vi "kinfe edge method.vi"(0 "Speed":cluster{"Speed":i32, "Vi":i32, "Vi steps":i32}={"Speed"=8000, "Vi"=1000, "Vi steps"=800} {"Speed" min=50 max=8000 step=50 scale=50.0..8000.0}, 1 "Go_stop":bool, 2 "PosCtrl":T2={"Go x"=FALSE, "Back x"=FALSE, "Go y"=FALSE, "Back y"=FALSE, "Go z"=FALSE, "Back z"=FALSE, "dX (um)"=1000, "dY (um)"=0, "dZ (um)"=0} {"dX (um)" step=1}, 5 "Home":bool, 7 "Zero":bool, 10 "stop 2":bool, 11 "VISA resource (RS232)":refnum<visa-resource-name>="COM1") -> (3 "?":cluster{"X":dbl, "Y":dbl, "Z":dbl}, 9 "Static":bool)   [LabVIEW 2014]
uses:
  <vilib>/vision/driver/NI_Vision_Acquisition_Software.lvlib
  <vilib>/Instr/_visa.llb/VISA Configure Serial Port (Instr).vi
  <vilib>/userdefined/High Color/IMAQdx.ctl
panel:
  out "um/s":string
  out "um(x) 2":string
  out "um(y)":string
  out "appended array":dbl[](array[numeric])
  out "fitting (y&T)":dbl[][](array[numeric])
  out "path (for logistic)":path
  out "row data save path":path
  in  "cluster":cluster{"T&Y(output)":dbl[][], "dt":dbl} {"dt" format="%#_13g"}
  out "T&Y(output)":dbl[][](array[numeric])
  out "Y(output)":dbl[](array[numeric])
  out "T(output)":dbl[](array[numeric])
  out "Initial X":dbl format="%^.3e"
  out "X Increment":dbl format="%^.3e"
  out "Y(all)":dbl[](array[numeric]) caption="Waveform Array" format="%^.3e"
  out "T(all)":dbl[](array[numeric])
  in  "Tout":i32
  in  "timeout":i32=5000 caption="Timeout\n[ms]"
  out "Waveform":T1(graph)
  out "Acquisitions":i32
  in  "Tab Control 2":enum32{"MAIN", "knife edge method", "Setting"}(tab)
  in  "?":enum32{" RS232", "ESP32"}(tab)
  in  "x-":bool caption="Start"
  in  "x+":bool caption="Start"
  out "um(x)":string
  in  "y+":bool caption="Start"
  in  "y-":bool caption="Start"
  in  "um":i32
  in  "um":i32
  in  "Channel":i32[](array[ring]) caption="Channel (1)" items=["1"=1, "2"=2, "3"=3, "4"=4, "off"=0]
  in  "?":bool
  in  "Get Image":bool
  out "Snap Image":T3(plugin-control)
  out "Grab Image":T3(plugin-control)
  in  "?":T4(tab)
  out "waveform 1":cluster{"T":dbl[], "Waveform Array":dbl[]}(graph)
  in  "unit":u16(ring) items=["s"=0, "ms"=3, "us"=6, "ns"=9]
  out "test read":dbl[](array[numeric])
  out "times":i32
  out "row data1":dbl[](array[numeric])
  out "row data1 2":dbl[](array[numeric])
  in  "Paramter guess":dbl[](array[numeric])=[-4.2, 0.0, 100.0, 1.0, 1.0]
  out "output cluster 2":T5
  out "waveform 2":cluster{"T":dbl[], "Waveform Array":dbl[]}(graph)
  in  "Save data":bool caption="Fitting"
  out "output cluster":T6
  in  "Slide":cluster{dbl, dbl}(slide)={0.0, 1.2121212121212122} scale=-0.9999920000000001..1.0000059999741622
  in  "name":string
  in  "Path":path
  out "XY Graph":cluster{cdb[]}[](graph)
  out "E":i32
  in  "fitting(Logistic)":bool caption="Fitting"
  in  "save(Logistic)":bool caption="Fitting"
  out "point":i32
  out "waveform 1":cluster{"T":dbl[], "Waveform Array":dbl[]}(graph)
  out "Samples count":i32[](array[numeric])
  in  "Exit":bool
  in  "Stop":bool
  in  "Single":bool
  in  "Start":bool
  out "ActiveChannels":i32[](array[numeric])=[1, 4]
  in  "channel on":i32=1 min=1 max=4 step=1
  in  "speed(um/s)":i32
  in  "move(um)":i32
  in  "knife edge method":bool caption="Start"
  in  "knife edge method(stop)":bool caption="Start"
  in  "VISA resource name 2":refnum<visa-resource-name>="TCPIP0::169.254.236.131::inst0::INSTR" caption="VISA resource name"
  in  "VISA resource name":refnum<visa-resource-name>="TCPIP::169.254.236.131::HISLIP"
  out "Moving Time (Sec)":dbl
  in  "VISA resource (esp32)":refnum<visa-resource-name>="COM8"
  in  "Delay (ms)":u32=100
  in  "update period (ms)":u32=100
  in  "Go":bool
  in  "Back":bool
  in  "X0":T7 {"Y (um)" min=0.0; "X (um)" min=0.0}
  in  "Scaling":cluster{"X":u16, "Y":u16, "Z":u16} {"Z" items=["X", "Z", "None"]; "Y" items=["X", "Z", "None"]; "X" items=["X", "Z", "None"]}
  in  "Position to go":T8={"Position"={"X"=FALSE, "Target X (um)"=1000.0, "Current X (um)"=1000.0, "Scaling X"=0, "Y"=FALSE, "Target Y (um)"=0.0, "Current Y (um)"=0.0, "Scaling Y"=0, "Z"=FALSE, "Target Z (um)"=0.0, "Current Z (um)"=0.0, "Scaling Z"=0}, "Speed"={"Speed"=3111, "Vi steps"=800, "Vi"=1000}} {"Speed"."Speed" min=50 max=8000 step=50 scale=50.0..8000.0; "Position"."Current X (um)" step=1.0; "Position"."Scaling Z" items=["X", "Z", "None"]; "Position"."Scaling Y" items=["X", "Z", "None"]; "Position"."Scaling X" items=["X", "Z", "None"]; "Position"."Target X (um)" step=1.0}
  in  "Camera COM":T9
  out "Position Info":T10={"Current coordinates"={"Steps"=0.0, "X"=FALSE, "Steps 2"=0.0, "Y"=FALSE, "Steps 3"=0.0, "Z"=FALSE}, "read buffer"="", "Command"="a", "Current coordinates 2"={"X"=0.0, "Y"=0.0, "Z"=0.0}, "Moving Time (Sec)"=0.0}
  out "RS232 error":errorcluster
  # "Only For Knife Edge Method"
  # "y0\n\nx0\n\nK\n\nL\n\nA"
  # "Esp32"
  # "CCD"
  # "RTO"
  # "RS232"
  # "Origin"
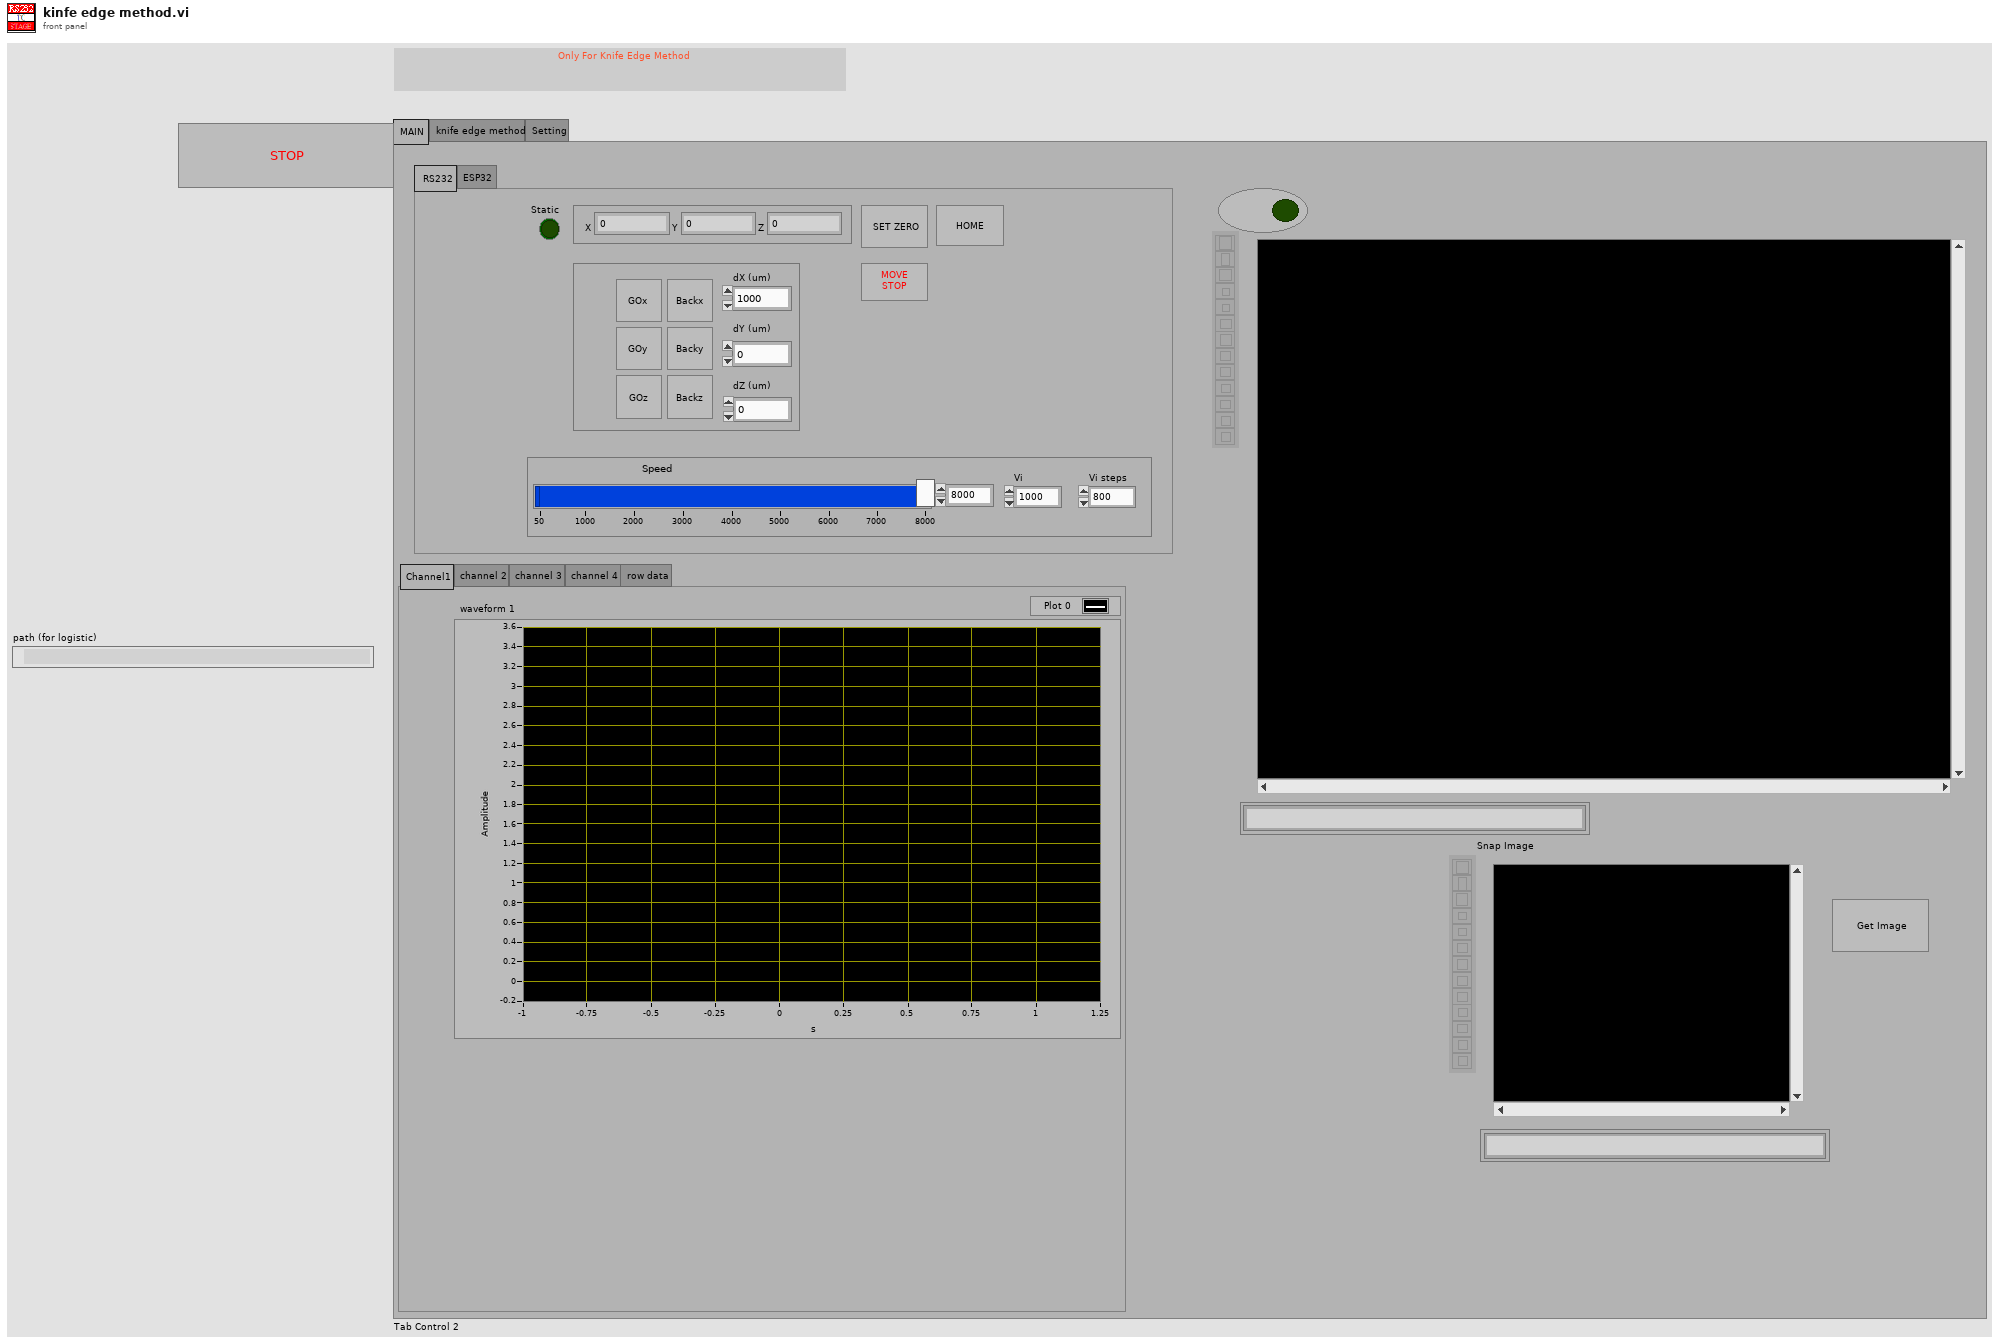
[diagram p1: front panel]
types:
  T1 = cluster{"Initial X":dbl, "X Increment":dbl, "Waveform Array":dbl[]}[]
  T2 = cluster{"Go x":bool, "Back x":bool, "Go y":bool, "Back y":bool, "Go z":bool, "Back z":bool, "dX (um)":u32, "dY (um)":u32, "dZ (um)":u32}
  T3 = typedef "IMAQ Image.ctl" = refnum<image>
  T4 = enum32{"Channel1", "channel 2", "channel 3", "channel 4", "row data"}
  T5 = cluster{"y0":dbl, "x0":dbl, "best fit parameters":dbl[]}
  T6 = cluster{"T(all)":dbl[], "Y(all)":dbl[], "X Increment":dbl, "Initial X":dbl}
  T7 = cluster{"X (um)":dbl, "X 2":bool, "Y (um)":dbl, "Y 2":bool, "Z (um)":dbl, "Z 2":bool}
  T8 = cluster{"Position":cluster{"X":bool, "Target X (um)":dbl, "Current X (um)":dbl, "Scaling X":u16, "Y":bool, "Target Y (um)":dbl, "Current Y (um)":dbl, "Scaling Y":u16, "Z":bool, "Target Z (um)":dbl, "Current Z (um)":dbl, "Scaling Z":u16}, "Speed":cluster{"Speed":i32, "Vi steps":i32, "Vi":i32}}
  T9 = typedef "IMAQdx.ctl" = refnum<k21>
  T10 = cluster{"Current coordinates":cluster{"Steps":dbl, "X":bool, "Steps 2":dbl, "Y":bool, "Steps 3":dbl, "Z":bool}, "read buffer":string, "Command":string, "Current coordinates 2":cluster{"X":dbl, "Y":dbl, "Z":dbl}, "Moving Time (Sec)":dbl}
  T11 = cluster{"X":bool, "Target X (um)":dbl, "Current X (um)":dbl, "Scaling X":u16, "Y":bool, "Target Y (um)":dbl, "Current Y (um)":dbl, "Scaling Y":u16, "Z":bool, "Target Z (um)":dbl, "Current Z (um)":dbl, "Scaling Z":u16}
  T12 = cluster{"Go x":bool, "Back x":bool, "Go y":bool, "Back y":bool, "Go z":bool, "Back z":bool, "dX (um)":dbl, "dY (um)":dbl, "dZ (um)":dbl}
  T13 = cluster{"Position":cluster{"X":bool, "Target X (um)":dbl, "Current X (um)":dbl, "Scaling X":u16, "Y":bool, "Target Y (um)":dbl, "Current Y (um)":dbl, "Scaling Y":u16, "Z":bool, "Target Z (um)":dbl, "Current Z (um)":dbl, "Scaling Z":u16}, "Value":cluster{"Speed":i32, "Vi":i32, "Vi steps":i32}}
  T14 = cluster{"Task":u16, cluster{"Position":cluster{"X":bool, "Target X (um)":dbl, "Current X (um)":dbl, "Scaling X":u16, "Y":bool, "Target Y (um)":dbl, "Current Y (um)":dbl, "Scaling Y":u16, "Z":bool, "Target Z (um)":dbl, "Current Z (um)":dbl, "Scaling Z":u16}, "Value":cluster{"Speed":i32, "Vi":i32, "Vi steps":i32}}}
  T15 = cluster{"Task":u16, "Position to go":cluster{"Position":cluster{"X":bool, "Target X (um)":dbl, "Current X (um)":dbl, "Scaling X":u16, "Y":bool, "Target Y (um)":dbl, "Current Y (um)":dbl, "Scaling Y":u16, "Z":bool, "Target Z (um)":dbl, "Current Z (um)":dbl, "Scaling Z":u16}, "Speed":cluster{"Speed":i32, "Vi steps":i32, "Vi":i32}}}
  T16 = cluster{"Task 2":u16, "Position to go 2":cluster{"Position":cluster{"X":bool, "Target X (um)":dbl, "Current X (um)":dbl, "Scaling X":u16, "Y":bool, "Target Y (um)":dbl, "Current Y (um)":dbl, "Scaling Y":u16, "Z":bool, "Target Z (um)":dbl, "Current Z (um)":dbl, "Scaling Z":u16}, "Speed":cluster{"Speed":i32, "Vi steps":i32, "Vi":i32}}}
  T17 = cluster{"Go x":bool, "Back x":bool, "Go y":bool, "Back y":bool, "Go z":bool, "Back z":bool, "dX (um)":bool, "dY (um)":bool, "dZ (um)":bool}
  T18 = cluster{"Initial X":dbl, "X Increment":dbl, "Waveform Array":dbl[]}
  T19 = cluster{"Ring":u16, "Value":cluster{"Position":cluster{"X":bool, "Target X (um)":dbl, "Current X (um)":dbl, "Scaling X":u16, "Y":bool, "Target Y (um)":dbl, "Current Y (um)":dbl, "Scaling Y":u16, "Z":bool, "Target Z (um)":dbl, "Current Z (um)":dbl, "Scaling Z":u16}, "Speed":cluster{"Speed":i32, "Vi steps":i32, "Vi":i32}}}
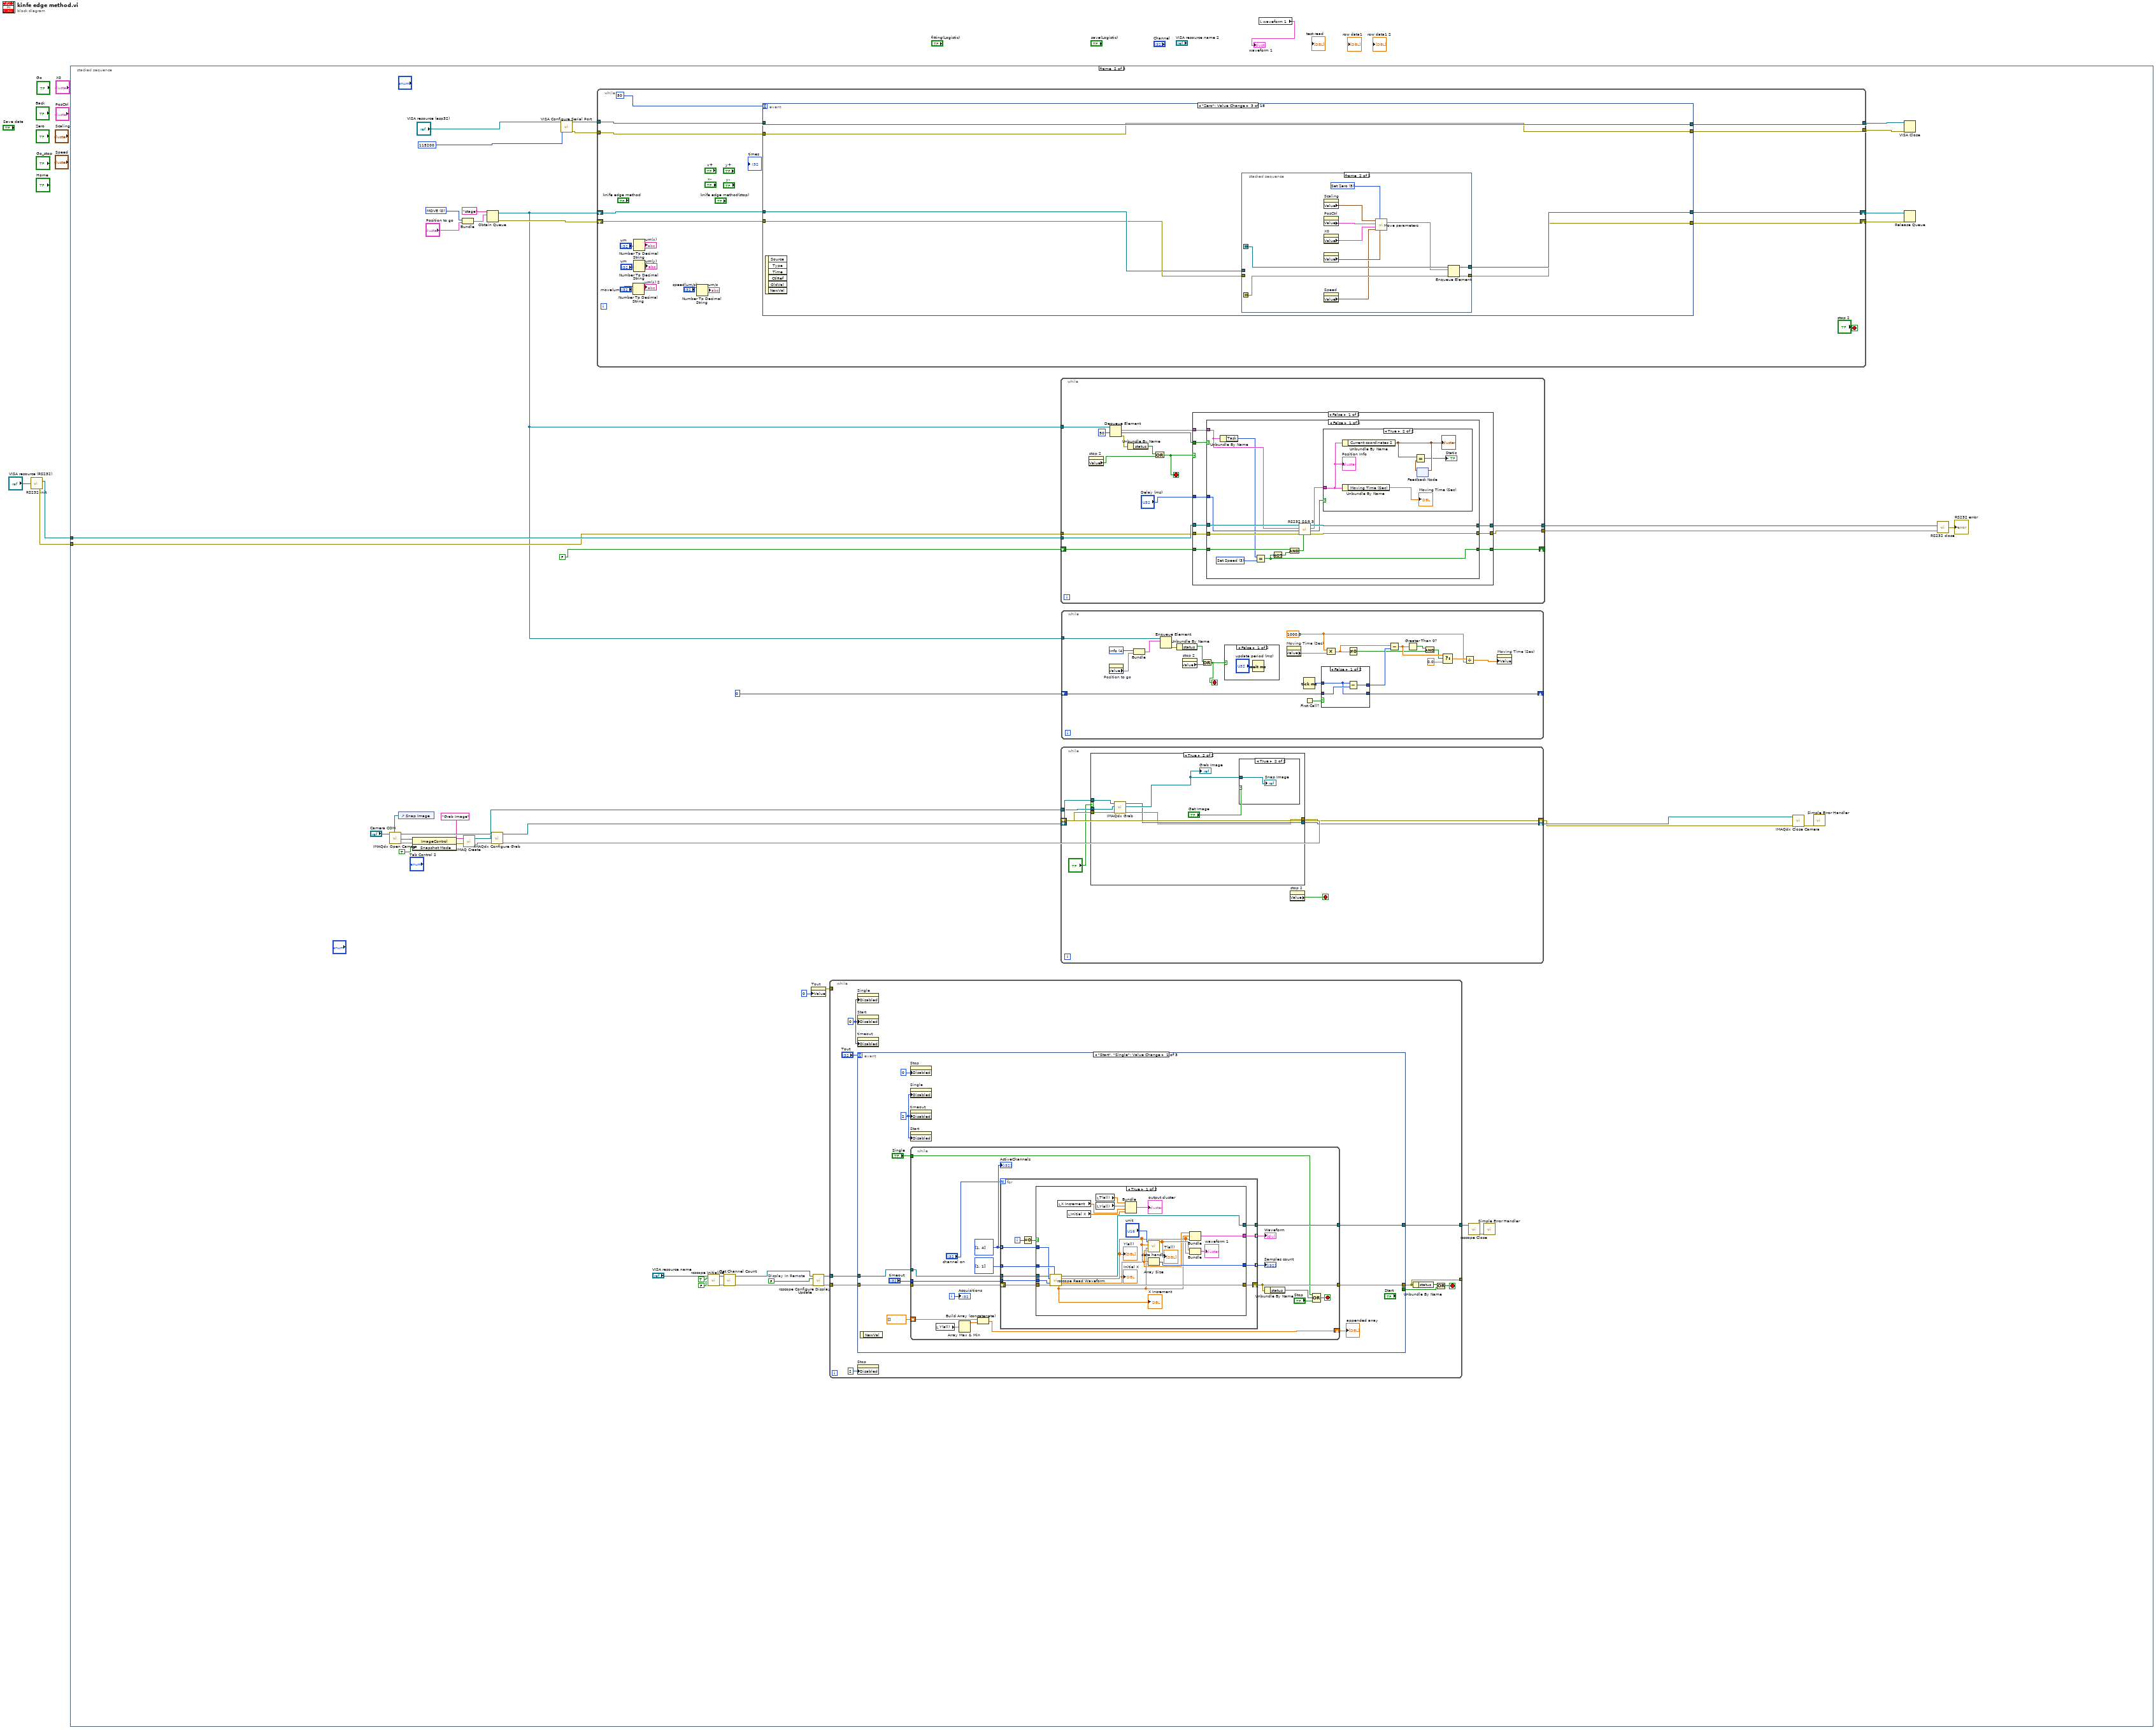
[diagram p0: block diagram]
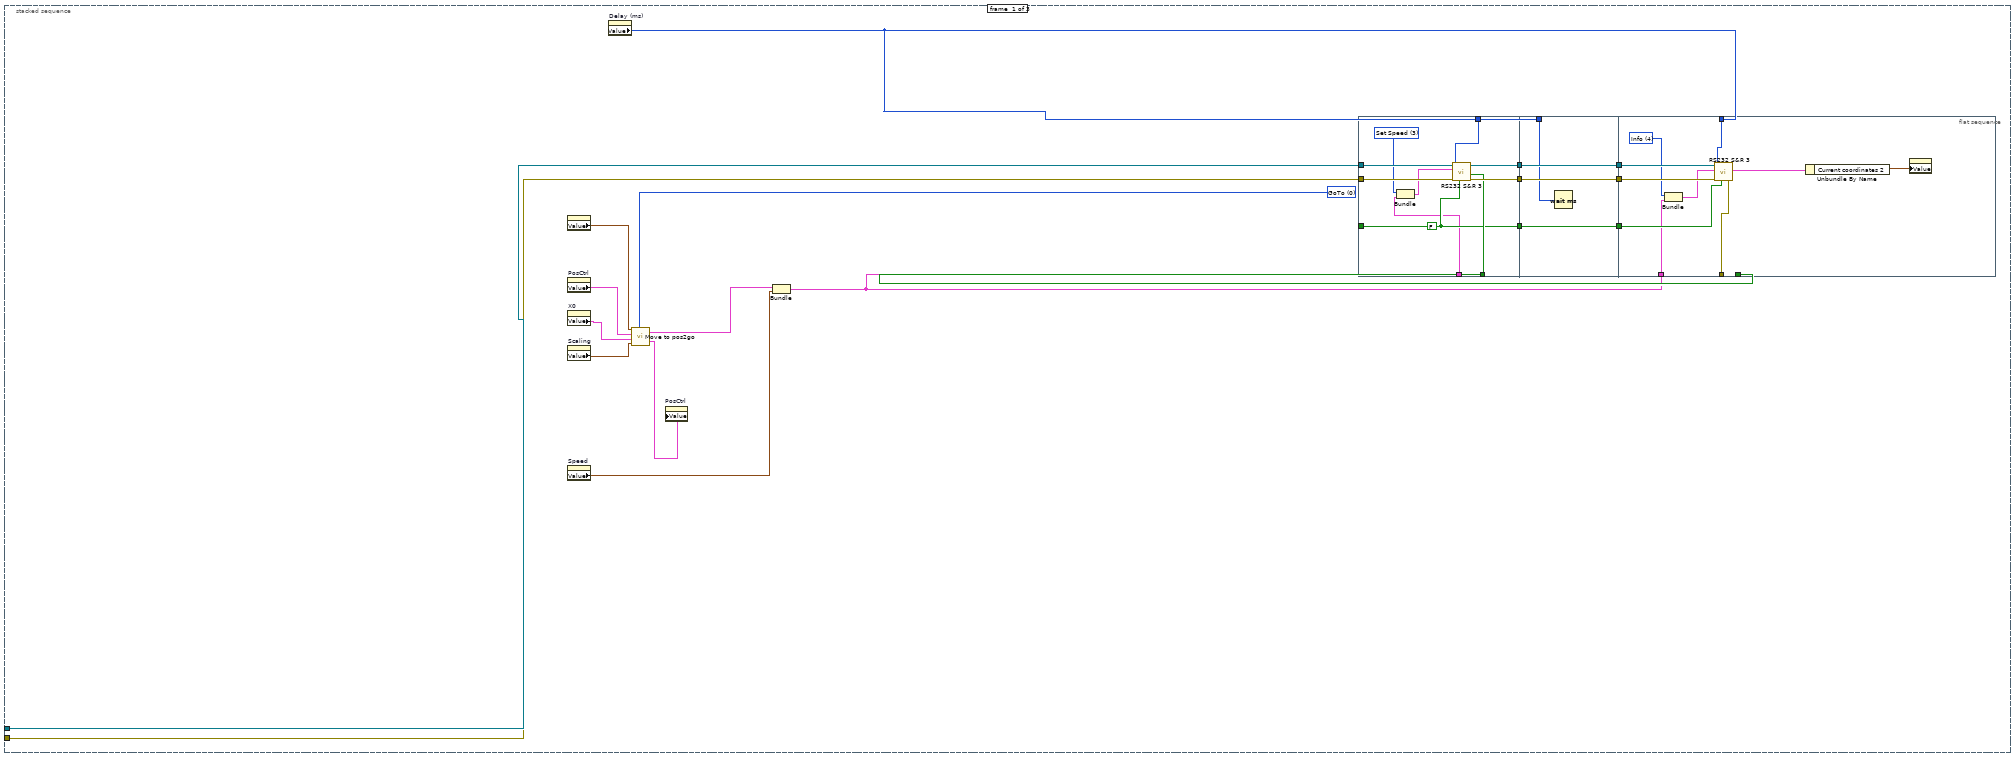
[diagram p2: hidden frame]
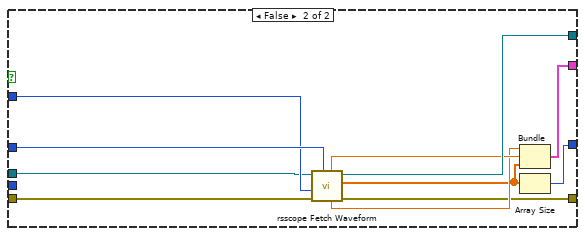
[diagram p3: hidden frame]
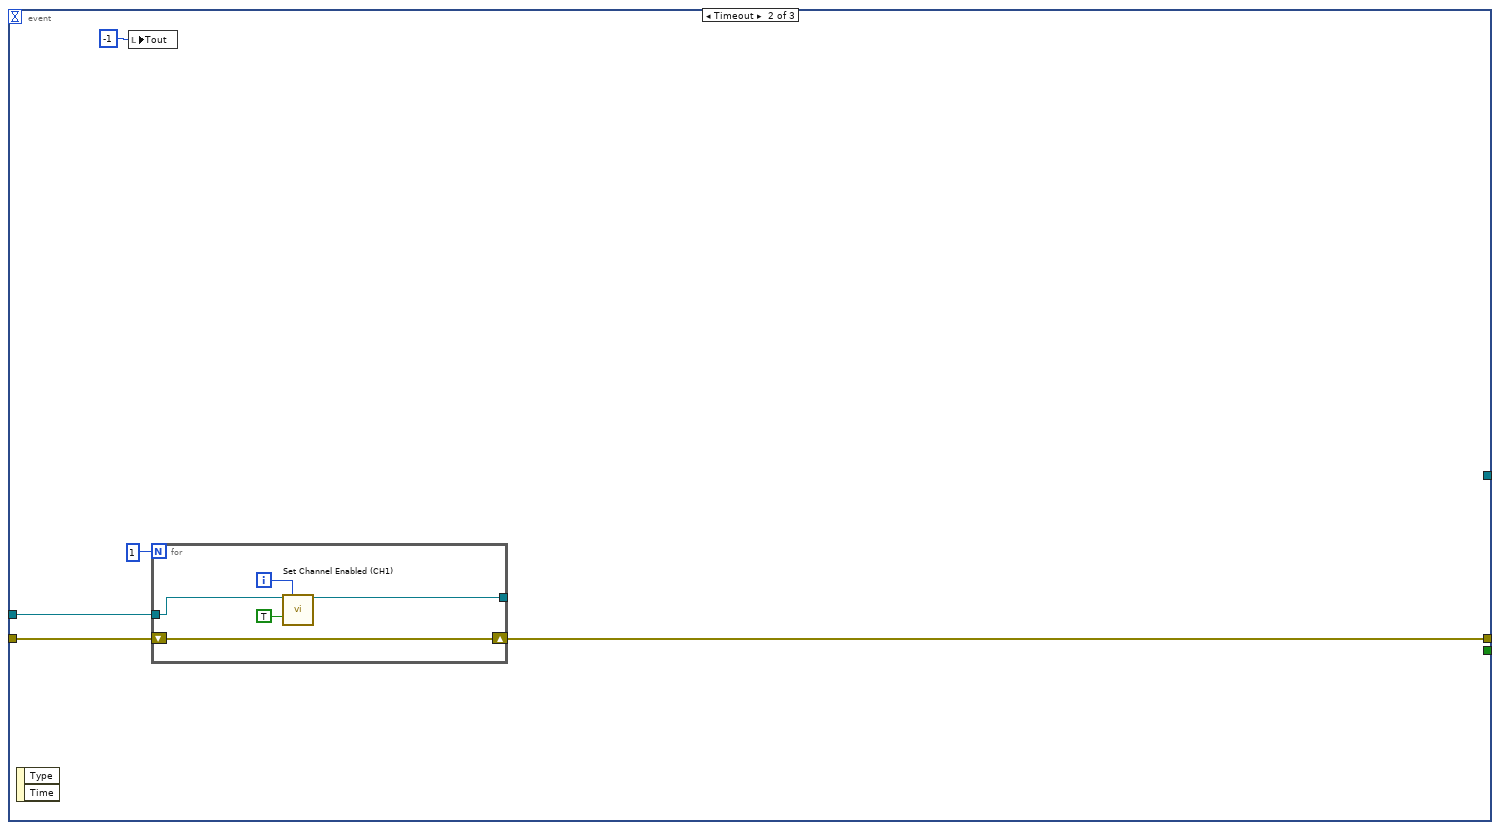
[diagram p4: hidden frame]
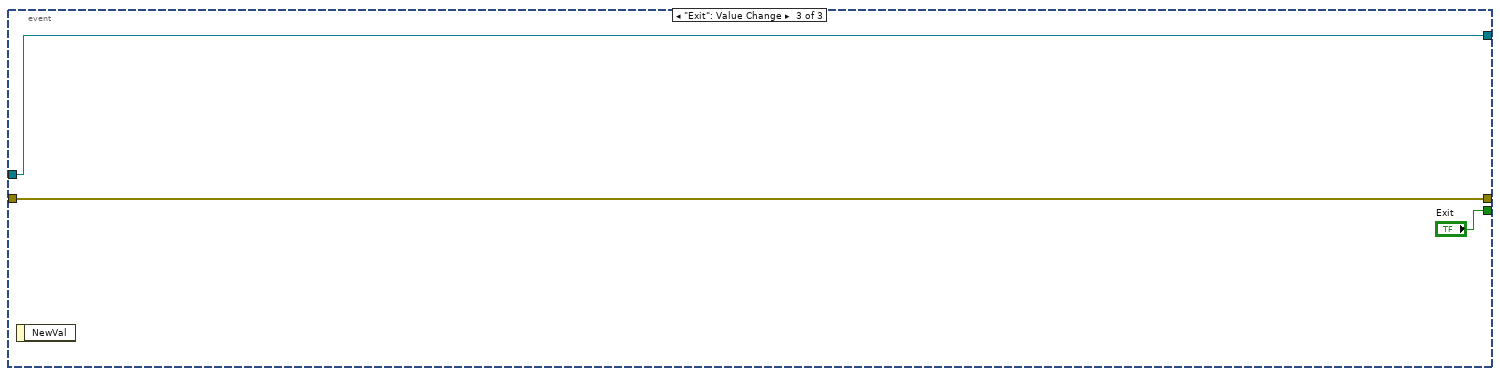
[diagram p5: hidden frame]
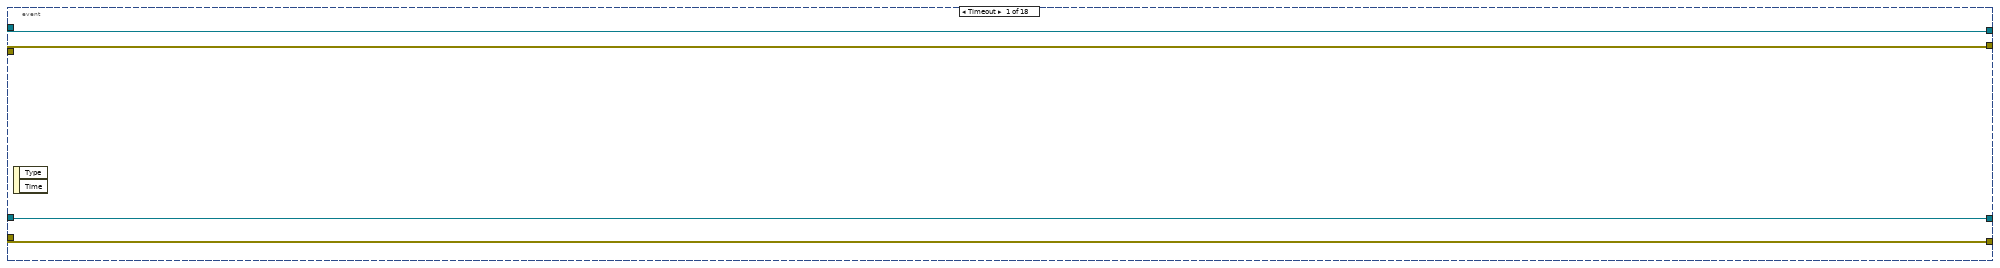
[diagram p13: hidden frame]
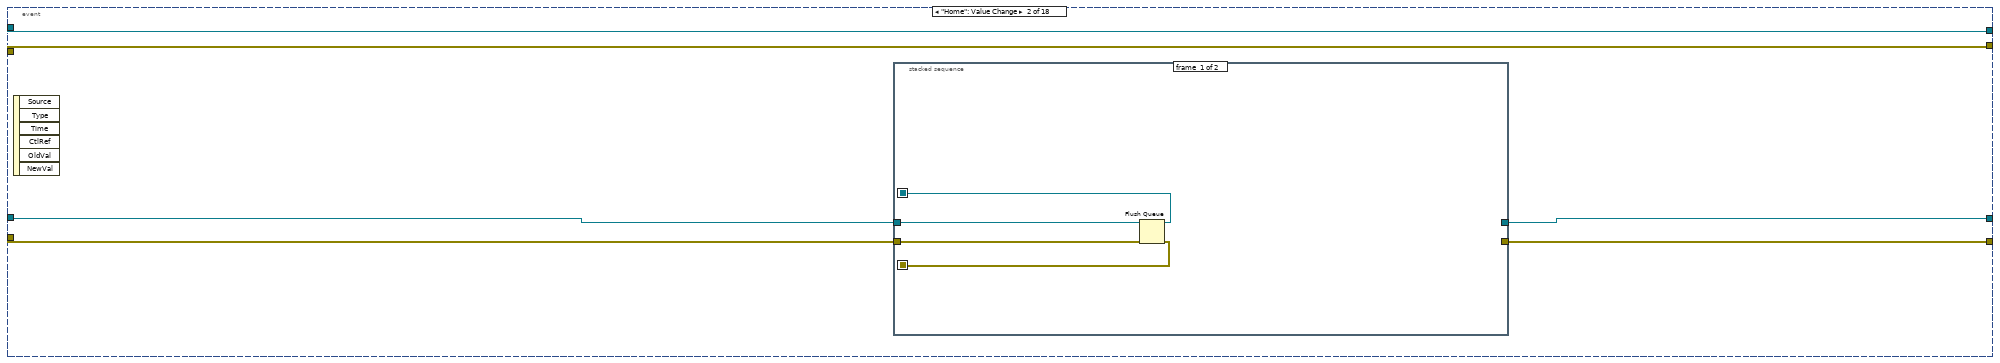
[diagram p14: hidden frame]
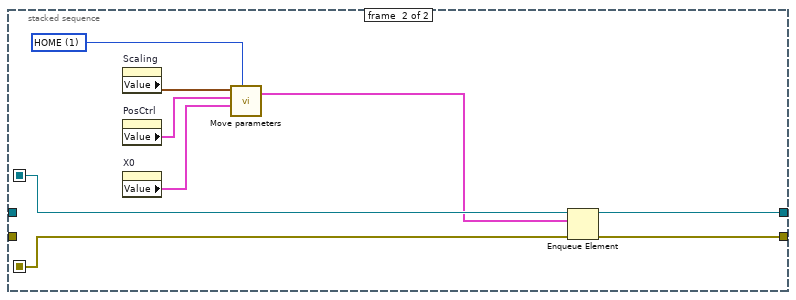
[diagram p15: hidden frame]
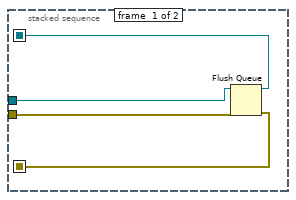
[diagram p16: hidden frame]
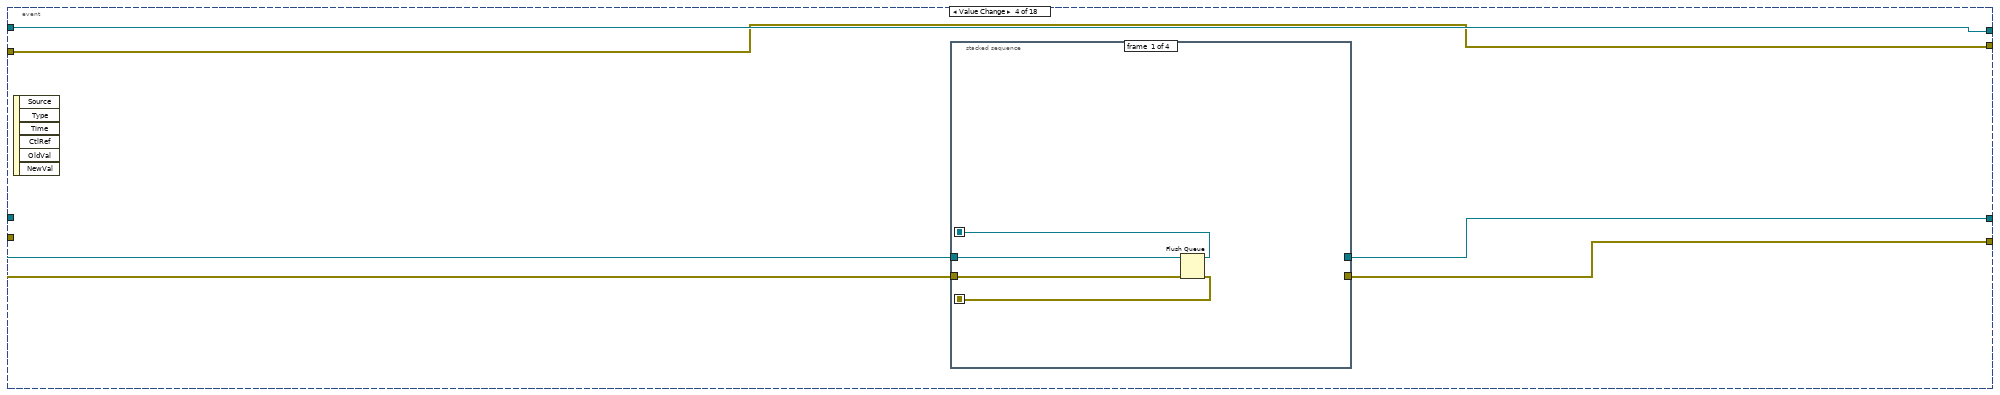
[diagram p17: hidden frame]
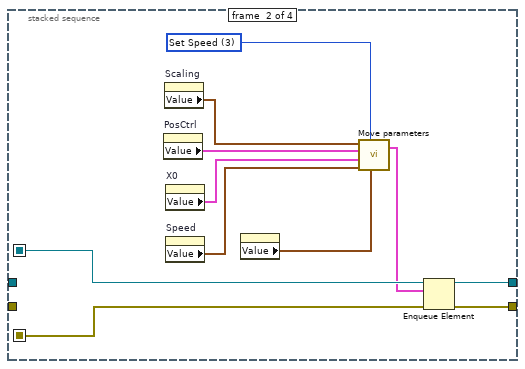
[diagram p18: hidden frame]
diagram:
  n1 = call "RS232 init.vi"("VISA resource name"="VISA resource (RS232)") -> ("VISA resource name out"=w3:refnum<visa-resource-name>, "error out"=w2:errorcluster)
  n2 = stacked-sequence {
    tunnel: w3 -> [w6 w90 _]
    tunnel: w2 -> [w5 w89 _]
    frame #0 {
      w11 = u16 0 items=["GoTo", "Jog"] ("Mode")
      n3 = property class="Clust (strict)"() -> ("Value"=w14:cluster{"X":dbl, "Y":dbl, "Z":dbl})  [unwired: 2 in, 2 out]
      n4 = property on="PosCtrl" class="Clust (strict)"() -> ("Value"=w13:T2)  [unwired: 2 in, 2 out]
      n5 = property on="X0" class="Clust (strict)"() -> ("Value"=w7:T7)  [unwired: 2 in, 2 out]
      n6 = property on="Scaling" class="Clust (strict)"() -> ("Value"=w12:cluster{"X":u16, "Y":u16, "Z":u16})  [unwired: 2 in, 2 out]
      n7 = property on="Speed" class="Clust (strict)"() -> ("Value"=w9:cluster{"Speed":i32, "Vi":i32, "Vi steps":i32})  [unwired: 2 in, 2 out]
      n8 = property on="Delay (ms)" class="DigNum (strict)"() -> ("Value"=w18:u32)  [unwired: 2 in, 2 out]
      n9 = call "Move to pos2go.vi"("Current coordinates"=w14, "DelX"=w13, "X0"=w7, "Scaling"=w12, "Mode"=w11) -> ("Position"=w10:T11, "DelX 2"=w8:T12)
      n10 = property on="PosCtrl" class="Clust (strict)"("Value"=w8) -> ()  [unwired: 2 in, 2 out]
      n11 = Bundle("Position"=w10, "Value"=w9) -> (w15:T13)  [unwired: 1 in]
      n12 = flat-sequence {
        tunnel: w6 -> [w34]
        tunnel: w5 -> [w33]
        tunnel: [w29] -> w16
        tunnel: w15 -> [w26]
        tunnel: [w32] -> w24
        tunnel: [w31] -> w23
        tunnel: w18 -> [w30]
        tunnel: FALSE -> [w28]
        tunnel: [w28] -> w22
        tunnel: [w38] -> w21
        tunnel: w24 -> [w38]
        tunnel: [w37] -> w20
        tunnel: w23 -> [w37]
        tunnel: w18 -> [w36]
        tunnel: [w35] -> w19
        tunnel: w22 -> [w35]
        tunnel: w21 -> [w48]
        tunnel: w20 -> [w47]
        tunnel: w18 -> [w46]
        tunnel: [w44] -> _
        tunnel: w16 -> [_]
        tunnel: w19 -> [w43]
        tunnel: w15 -> [w41]
        frame #0 {
          w27 = u16 3 items=["MOVE", "HOME", "STOP", "Set Speed", "Info", "Set Zero"] ("Task")
          n13 = Bundle("Task"=w27, w26) -> (w25:T14)  [unwired: 1 in]
          n14 = call "RS232 S&R 3.vi"("ReSetSPD"=w28, "error in"=w33, "Delay (ms)"=w30, "Stage Control"=w25, "VISA resource in"=w34) -> ("error out"=w31:errorcluster, "read"=w29:bool, "VISA resource name out"=w32:refnum<visa-resource-name>)  [unwired: 1 out]
        }
        frame #1 {
          n15 = Wait (ms)(milliseconds to wait=w36) -> ()  [unwired: 1 out]
        }
        frame #2 {
          w40 = u16 4 items=["MOVE", "HOME", "STOP", "Set Speed", "Info", "Set Zero"] ("Task")
          n16 = Bundle("Task"=w40, w41) -> (w39:T14)  [unwired: 1 in]
          n17 = call "RS232 S&R 3.vi"("ReSetSPD"=w43, "error in"=w47, "Delay (ms)"=w46, "Stage Control"=w39, "VISA resource in"=w48) -> ("error out"=w44:errorcluster, "Cluster"=w42:T10)  [unwired: 2 out]
          n18 = Unbundle By Name(w42) -> ("Current coordinates 2"=w45:cluster{"X":dbl, "Y":dbl, "Z":dbl})
          n19 = property class="Clust (strict)"("Value"=w45) -> ()  [unwired: 2 in, 2 out]
        }
      }
    }
    frame #1 {
      w55 = FALSE  # Display In Remote
      w95 = u16 0 items=["MOVE", "HOME", "STOP", "Set Speed", "Info", "Set Zero", "MOVE2"] ("Task")
      n20 = call <vilib>:"IMAQdx Open Camera.vi"("Session In"="Camera COM") -> ("error out"=w75:errorcluster, "Session Out"=w74:T9)  [unwired: 2 in, 7 out]
      n21 = control-ref of="Snap Image"() -> (w76:refnum<vi>)
      n22 = property class="ImageControl"(reference=w76, error in=w75, "Snapshot Mode"=TRUE) -> (error out=w73:errorcluster)  [unwired: 1 out]
      n23 = Bundle("Task"=w95, "Position to go"="Position to go") -> (w96:T15)  [unwired: 1 in]
      n24 = call "IMAQ Create"("Image Name"="Grab Image", "error in (no error)"=w73) -> ("New Image"=w63:T3, "error out"=w72:errorcluster)  [unwired: 2 in, 1 out]
      n25 = Obtain Queue(name (unnamed)="stage", element data type=w96) -> (queue out=w84:refnum<queue>, error out=w93:errorcluster)  [unwired: 3 in, 1 out]
      n26 = call <vilib>:"IMAQdx Configure Grab.vi"("error in"=w72, "Session In"=w74) -> ("error out"=w65:errorcluster, "Session Out"=w64:T9)  [unwired: 8 out]
      n27 = call-poly "VISA Configure Serial Port"("VISA resource name"="VISA resource (esp32)", "baud rate (9600)"=u32 115200) -> ("VISA resource name out"=w80:refnum<visa-resource-name>, "error out"=w79:errorcluster)  [unwired: 12 in]
      n28 = while {
        shift-right: [w301] -> w92
        shift-left: w84 -> [w304]
        shift-right: [w300] -> w91
        shift-left: w93 -> [w303]
        tunnel: w80 -> [w287]
        tunnel: w79 -> [w288]
        tunnel: [w299] -> w78
        tunnel: [w298] -> w77
        stop <- "stop 2" stop-if-true
        n29 = Number To Decimal String(number="move(um)") -> (decimal integer string=→"um(x) 2":string)  [unwired: 1 in]
        n30 = Number To Decimal String(number="um") -> (decimal integer string=→"um(x)":string)  [unwired: 1 in]
        n31 = Number To Decimal String(number="um") -> (decimal integer string=→"um(y)":string)  [unwired: 1 in]
        n32 = Number To Decimal String(number="speed(um/s)") -> (decimal integer string=→"um/s":string)  [unwired: 1 in]
        n33 = event shown="[2] \"Zero\": Value Change" {
          selector: _ -> [_ _ _ _ _ _ _ _ _ _ _ _ _ _ _ _ _ _]
          dyn-events: _ -> [_ _ _ _ _ _ _ _ _ _ _ _ _ _ _ _ _ _]
          timeout: 50 -> [_ _ _ _ _ _ _ _ _ _ _ _ _ _ _ _ _ _]
          tunnel: w304 -> [w308 w314 w333 w354 w375 w396 w417 w438 w481 w495 w503 w514 w522 w532 w542 w553 w564 w574]
          tunnel: w303 -> [w307 w313 w332 w353 w374 w395 w416 w437 w480 w494 w502 w513 w521 w531 w541 w552 w563 w573]
          tunnel: [w308 w312 w331 w352 w373 w394 w415 w436 w481 w495 w503 w514 w522 w532 w542 w553 w564 w574] -> w301
          tunnel: [w307 w311 w330 w351 w372 w393 w414 w435 w480 w494 w502 w513 w521 w531 w541 w552 w563 w573] -> w300
          tunnel: w287 -> [w306 w310 w329 w350 w371 w392 w413 w434 w483 w497 w505 w516 w526 w536 w546 w557 w568 w576]
          tunnel: w288 -> [w305 w309 w328 w349 w370 w391 w412 w433 w482 w496 w504 w515 w525 w535 w545 w556 w567 w575]
          tunnel: [w306 w310 w329 w350 w371 w392 w413 w434 w483 w497 w505 w516 w524 w534 w544 w555 w562 w572] -> w299
          tunnel: [w305 w309 w328 w349 w370 w391 w412 w433 w482 w496 w504 w515 w523 w533 w543 w554 w561 w571] -> w298
          event Timeout {
            n34 = event-data() -> ()  [unwired: 1 in, 2 out]
          }
          event "Home": Value Change {
            n35 = event-data() -> ()  [unwired: 1 in, 6 out]
            n36 = stacked-sequence {
              seq-local: [w315 _] -> [_ w325]
              seq-local: [w316 _] -> [_ w324]
              tunnel: w314 -> [w318 _]
              tunnel: w313 -> [w317 _]
              tunnel: [_ w327] -> w312
              tunnel: [_ w326] -> w311
              frame #0 {
                n37 = Flush Queue(queue=w318, error in (no error)=w317) -> (queue out=w315:refnum<queue>, error out=w316:errorcluster)  [unwired: 1 out]
              }
              frame #1 {
                w320 = u16 1 items=["MOVE", "HOME", "ZERO", "Set speed", "Info"] ("Ring")
                n38 = property on="Scaling" class="Clust (strict)"() -> ("Value"=w323:cluster{"X":u16, "Y":u16, "Z":u16})  [unwired: 2 in, 2 out]
                n39 = property on="PosCtrl" class="Clust (strict)"() -> ("Value"=w322:T2)  [unwired: 2 in, 2 out]
                n40 = property on="X0" class="Clust (strict)"() -> ("Value"=w319:T7)  [unwired: 2 in, 2 out]
                n41 = call "Move parameters.vi"("Task"=w320, "X0"=w319, "PosCtrl"=w322, "Scaling"=w323) -> ("Move info"=w321:T16)  [unwired: 2 in, 1 out]
                n42 = Enqueue Element(queue=w325, element=w321, error in (no error)=w324) -> (queue out=w327:refnum<queue>, error out=w326:errorcluster)  [unwired: 1 in, 1 out]
              }
            }
          }
          event "Zero": Value Change {
            n43 = event-data() -> ()  [unwired: 1 in, 6 out]
            n44 = stacked-sequence {
              seq-local: [w335 _] -> [_ w348]
              seq-local: [w336 _] -> [_ w347]
              tunnel: w332 -> [w337 _]
              tunnel: [_ w346] -> w331
              tunnel: [_ w345] -> w330
              tunnel: w333 -> [w334 _]
              frame #0 {
                n45 = Flush Queue(queue=w334, error in (no error)=w337) -> (queue out=w335:refnum<queue>, error out=w336:errorcluster)  [unwired: 1 out]
              }
              frame #1 {
                w344 = u16 5 items=["MOVE", "HOME", "STOP", "Set Speed", "Info", "Set Zero"] ("Task")
                n46 = property on="Scaling" class="Clust (strict)"() -> ("Value"=w342:cluster{"X":u16, "Y":u16, "Z":u16})  [unwired: 2 in, 2 out]
                n47 = property on="PosCtrl" class="Clust (strict)"() -> ("Value"=w341:T2)  [unwired: 2 in, 2 out]
                n48 = property on="X0" class="Clust (strict)"() -> ("Value"=w340:T7)  [unwired: 2 in, 2 out]
                n49 = property class="Clust (strict)"() -> ("Value"=w343:cluster{"X":dbl, "Y":dbl, "Z":dbl})  [unwired: 2 in, 2 out]
                n50 = property on="Speed" class="Clust (strict)"() -> ("Value"=w339:cluster{"Speed":i32, "Vi":i32, "Vi steps":i32})  [unwired: 2 in, 2 out]
                n51 = call "Move parameters.vi"("Current coordinates"=w343, "Task"=w344, "Speed"=w339, "X0"=w340, "PosCtrl"=w341, "Scaling"=w342) -> ("Move info"=w338:T16)  [unwired: 1 out]
                n52 = Enqueue Element(queue=w348, element=w338, error in (no error)=w347) -> (queue out=w346:refnum<queue>, error out=w345:errorcluster)  [unwired: 1 in, 1 out]
              }
            }
          }
          event "Speed.Speed": Value Change {
            n53 = event-data() -> ()  [unwired: 1 in, 6 out]
            n54 = stacked-sequence {
              seq-local: [w356 _ _ _] -> [_ w367 _ _]
              seq-local: [w355 _ _ _] -> [_ w366 _ _]
              tunnel: w354 -> [w358 _ _ _]
              tunnel: [_ w369 _ _] -> w352
              tunnel: w353 -> [w357 _ _ _]
              tunnel: [_ w368 _ _] -> w351
              frame #0 {
                n55 = Flush Queue(queue=w358, error in (no error)=w357) -> (queue out=w356:refnum<queue>, error out=w355:errorcluster)  [unwired: 1 out]
              }
              frame #1 {
                w365 = u16 3 items=["MOVE", "HOME", "STOP", "Set Speed", "Info", "Set Zero"] ("Task")
                n56 = property on="PosCtrl" class="Clust (strict)"() -> ("Value"=w363:T2)  [unwired: 2 in, 2 out]
                n57 = property on="Scaling" class="Clust (strict)"() -> ("Value"=w364:cluster{"X":u16, "Y":u16, "Z":u16})  [unwired: 2 in, 2 out]
                n58 = property on="X0" class="Clust (strict)"() -> ("Value"=w362:T7)  [unwired: 2 in, 2 out]
                n59 = property on="Speed" class="Clust (strict)"() -> ("Value"=w361:cluster{"Speed":i32, "Vi":i32, "Vi steps":i32})  [unwired: 2 in, 2 out]
                n60 = property class="Clust (strict)"() -> ("Value"=w360:cluster{"X":dbl, "Y":dbl, "Z":dbl})  [unwired: 2 in, 2 out]
                n61 = call "Move parameters.vi"("Current coordinates"=w360, "Task"=w365, "Speed"=w361, "X0"=w362, "PosCtrl"=w363, "Scaling"=w364) -> ("Move info"=w359:T16)  [unwired: 1 out]
                n62 = Enqueue Element(queue=w367, element=w359, error in (no error)=w366) -> (queue out=w369:refnum<queue>, error out=w368:errorcluster)  [unwired: 1 in, 1 out]
              }
              frame #2 {
              }
              frame #3 {
              }
            }
          }
          event "Go": Value Change {
            n63 = event-data() -> ()  [unwired: 1 in, 6 out]
            n64 = stacked-sequence {
              seq-local: [w376 _] -> [_ w388]
              seq-local: [w377 _] -> [_ w387]
              tunnel: w375 -> [w379 _]
              tunnel: w374 -> [w378 _]
              tunnel: [_ w390] -> w373
              tunnel: [_ w389] -> w372
              frame #0 {
                n65 = Flush Queue(queue=w379, error in (no error)=w378) -> (queue out=w376:refnum<queue>, error out=w377:errorcluster)  [unwired: 1 out]
              }
              frame #1 {
                w380 = u16 6 items=["MOVE", "HOME", "STOP", "Set Speed", "Info", "Set Zero", "MOVE2"] ("Task")
                n66 = property on="Scaling" class="Clust (strict)"() -> ("Value"=w384:cluster{"X":u16, "Y":u16, "Z":u16})  [unwired: 2 in, 2 out]
                n67 = property on="PosCtrl" class="Clust (strict)"() -> ("Value"=w385:T2)  [unwired: 2 in, 2 out]
                n68 = property on="X0" class="Clust (strict)"() -> ("Value"=w383:T7)  [unwired: 2 in, 2 out]
                n69 = property on="Speed" class="Clust (strict)"() -> ("Value"=w382:cluster{"Speed":i32, "Vi":i32, "Vi steps":i32})  [unwired: 2 in, 2 out]
                n70 = property class="Clust (strict)"() -> ("Value"=w381:cluster{"X":dbl, "Y":dbl, "Z":dbl})  [unwired: 2 in, 2 out]
                n71 = call "Move parameters.vi"("Current coordinates"=w381, "Task"=w380, "Speed"=w382, "X0"=w383, "PosCtrl"=w385, "Scaling"=w384) -> ("Move info"=w386:T16)  [unwired: 1 out]
                n72 = Enqueue Element(queue=w388, element=w386, error in (no error)=w387) -> (queue out=w390:refnum<queue>, error out=w389:errorcluster)  [unwired: 1 in, 1 out]
              }
            }
          }
          event "Back": Value Change {
            n73 = event-data() -> ()  [unwired: 1 in, 6 out]
            n74 = stacked-sequence {
              seq-local: [w397 _] -> [_ w409]
              seq-local: [w398 _] -> [_ w408]
              tunnel: w396 -> [w400 _]
              tunnel: w395 -> [w399 _]
              tunnel: [_ w411] -> w394
              tunnel: [_ w410] -> w393
              frame #0 {
                n75 = Flush Queue(queue=w400, error in (no error)=w399) -> (queue out=w397:refnum<queue>, error out=w398:errorcluster)  [unwired: 1 out]
              }
              frame #1 {
                w401 = u16 6 items=["MOVE", "HOME", "STOP", "Set Speed", "Info", "Set Zero", "MOVE2"] ("Task")
                n76 = property on="Scaling" class="Clust (strict)"() -> ("Value"=w405:cluster{"X":u16, "Y":u16, "Z":u16})  [unwired: 2 in, 2 out]
                n77 = property on="PosCtrl" class="Clust (strict)"() -> ("Value"=w406:T2)  [unwired: 2 in, 2 out]
                n78 = property on="X0" class="Clust (strict)"() -> ("Value"=w404:T7)  [unwired: 2 in, 2 out]
                n79 = property on="Speed" class="Clust (strict)"() -> ("Value"=w403:cluster{"Speed":i32, "Vi":i32, "Vi steps":i32})  [unwired: 2 in, 2 out]
                n80 = property class="Clust (strict)"() -> ("Value"=w402:cluster{"X":dbl, "Y":dbl, "Z":dbl})  [unwired: 2 in, 2 out]
                n81 = call "Move parameters.vi"("Current coordinates"=w402, "Task"=w401, "Speed"=w403, "X0"=w404, "PosCtrl"=w406, "Scaling"=w405) -> ("Move info"=w407:T16)  [unwired: 1 out]
                n82 = Enqueue Element(queue=w409, element=w407, error in (no error)=w408) -> (queue out=w411:refnum<queue>, error out=w410:errorcluster)  [unwired: 1 in, 1 out]
              }
            }
          }
          event "Go_stop": Value Change {
            n83 = event-data() -> ()  [unwired: 1 in, 6 out]
            n84 = stacked-sequence {
              seq-local: [w418 _] -> [_ w429]
              seq-local: [w419 _] -> [_ w430]
              tunnel: w417 -> [w421 _]
              tunnel: w416 -> [w420 _]
              tunnel: [_ w432] -> w415
              tunnel: [_ w431] -> w414
              frame #0 {
                n85 = Flush Queue(queue=w421, error in (no error)=w420) -> (queue out=w418:refnum<queue>, error out=w419:errorcluster)  [unwired: 1 out]
              }
              frame #1 {
                w428 = u16 2 items=["MOVE", "HOME", "STOP", "Set Speed", "Info", "Set Zero"] ("Task")
                n86 = property on="Scaling" class="Clust (strict)"() -> ("Value"=w427:cluster{"X":u16, "Y":u16, "Z":u16})  [unwired: 2 in, 2 out]
                n87 = property on="PosCtrl" class="Clust (strict)"() -> ("Value"=w426:T2)  [unwired: 2 in, 2 out]
                n88 = property on="X0" class="Clust (strict)"() -> ("Value"=w425:T7)  [unwired: 2 in, 2 out]
                n89 = property on="Speed" class="Clust (strict)"() -> ("Value"=w424:cluster{"Speed":i32, "Vi":i32, "Vi steps":i32})  [unwired: 2 in, 2 out]
                n90 = property class="Clust (strict)"() -> ("Value"=w423:cluster{"X":dbl, "Y":dbl, "Z":dbl})  [unwired: 2 in, 2 out]
                n91 = call "Move parameters.vi"("Current coordinates"=w423, "Task"=w428, "Speed"=w424, "X0"=w425, "PosCtrl"=w426, "Scaling"=w427) -> ("Move info"=w422:T16)  [unwired: 1 out]
                n92 = Enqueue Element(queue=w429, element=w422, error in (no error)=w430) -> (queue out=w432:refnum<queue>, error out=w431:errorcluster)  [unwired: 1 in, 1 out]
              }
            }
          }
          event "PosCtrl": Value Change {
            n93 = event-data() -> ("OldVal"=w441:T2, "NewVal"=w440:T2)  [unwired: 1 in, 4 out]
            n94 = Equal?(x=w441, y=w440) -> (x = y?=w448:T17)
            n95 = Unbundle By Name(w448) -> ("Go x"=w447:bool, "Back x"=w446:bool, "Go y"=w445:bool, "Back y"=w444:bool, "Go z"=w443:bool, "Back z"=w442:bool)
            n96 = Compound Arithmetic op=OR(w447, w446, w445, w444, w443, w442) -> (w439:bool)
            n97 = case shown="True" w439 {
              tunnel: [w450 w454] -> w436
              tunnel: [w449 w453] -> w435
              tunnel: w438 -> [w450 w452]
              tunnel: w437 -> [w449 w451]
              frame False {
              }
              frame True {
                n98 = stacked-sequence {
                  seq-local: [w455 _ _] -> [_ w467 _]
                  seq-local: [w456 _ _] -> [_ w468 _]
                  seq-local: [_ w459 _] -> [_ _ w471]
                  tunnel: w452 -> [w458 _ _]
                  tunnel: w451 -> [w457 _ _]
                  tunnel: [_ w470 _] -> w454
                  tunnel: [_ w469 _] -> w453
                  frame #0 {
                    n99 = Flush Queue(queue=w458, error in (no error)=w457) -> (queue out=w455:refnum<queue>, error out=w456:errorcluster)  [unwired: 1 out]
                  }
                  frame #1 {
                    w460 = u16 0 items=["MOVE", "HOME", "STOP", "Set Speed", "Info", "Set Zero", "MOVE2"] ("Task")
                    n100 = property on="Scaling" class="Clust (strict)"() -> ("Value"=w466:cluster{"X":u16, "Y":u16, "Z":u16})  [unwired: 2 in, 2 out]
                    n101 = property on="PosCtrl" class="Clust (strict)"() -> ("Value"=w465:T2)  [unwired: 2 in, 2 out]
                    n102 = property on="X0" class="Clust (strict)"() -> ("Value"=w464:T7)  [unwired: 2 in, 2 out]
                    n103 = property on="Speed" class="Clust (strict)"() -> ("Value"=w463:cluster{"Speed":i32, "Vi":i32, "Vi steps":i32})  [unwired: 2 in, 2 out]
                    n104 = property class="Clust (strict)"() -> ("Value"=w462:cluster{"X":dbl, "Y":dbl, "Z":dbl})  [unwired: 2 in, 2 out]
                    n105 = call "Move parameters.vi"("Current coordinates"=w462, "Task"=w460, "Speed"=w463, "X0"=w464, "PosCtrl"=w465, "Scaling"=w466) -> ("PosCtrl out"=w459:T12, "Move info"=w461:T16)
                    n106 = Enqueue Element(queue=w467, element=w461, error in (no error)=w468) -> (queue out=w470:refnum<queue>, error out=w469:errorcluster)  [unwired: 1 in, 1 out]
                  }
                  frame #2 {
                    n107 = property on="PosCtrl" class="Clust (strict)"("Value"=w471) -> ()  [unwired: 2 in, 2 out]
                  }
                }
              }
            }
          }
          event "Slide": Value Change {
            n108 = event-data() -> ()  [unwired: 1 in, 6 out]
            n109 = local read "T&Y(output)"() -> (w475:dbl[][])
            n110 = local read "X Increment"() -> (w477:dbl)
            n111 = Transpose 2D Array(2D array=w475) -> (transposed array=w474:dbl[][])
            n112 = Bundle(w474, "X Increment"=w477) -> (w476:cluster{dbl[][], "X Increment":dbl})  [unwired: 1 in]
            n113 = local read "output cluster"() -> (w492:T6)
            n114 = local write "cluster"(w476) -> ()
            n115 = Unbundle(w492) -> ("T(all)"=w491:dbl[], "Y(all)"=w490:dbl[], "X Increment"=w488:dbl, "Initial X"=w489:dbl)
            n116 = call "split data.vi"("Slide"="Slide", "dt"=w488, "t0"=w489, "Y(input)"=w490, "T(input)"=w491) -> ("max value"=w485:dbl, "min value"=w486:dbl, "Y(output)"=w473:dbl[], "T(output)"=w479:dbl[])  [unwired: 2 in]
            "T(output)" <- w479
            "Y(output)" <- w473
            n117 = property on="Slide" class="Slide (strict)"("Scale.Maximum"=w485, "Scale.Minimum"=w486) -> ()  [unwired: 2 in, 2 out]
            n118 = Bundle("T(output)"=w479, "Y(output)"=w473) -> (→"waveform 2":cluster{"T(output)":dbl[], "Y(output)":dbl[]})  [unwired: 1 in]
            n119 = Array Size(array=w473) -> (size(s)=→"point":i32)
            n120 = Build Array(w479, w473) -> (→"T&Y(output)":dbl[][])
          }
          event "Save data": Value Change {
            n121 = event-data() -> ()  [unwired: 1 in, 6 out]
            n122 = call "save data.vi"("name"="name", "Path"="Path", "cluster"="cluster") -> ("new file path (Not A Path if cancelled)"=→"row data save path":path, "path(FOR logistic"=→"path (for logistic)":path)  [unwired: 6 in, 1 out]
          }
          event "fitting(Logistic)": Value Change {
            n123 = event-data() -> ()  [unwired: 1 in, 6 out]
            n124 = local read "Y(output)"() -> (w511:dbl[])
            n125 = local read "T(output)"() -> (w512:dbl[])
            n126 = call "Fittinglogistic_MODCA.vi"("Paramter guess"="Paramter guess", "y"=w511, "t"=w512) -> ("fitting (y&T)"=→"fitting (y&T)":dbl[][], "E"=→"E":i32, "XY Graph"=→"XY Graph":cluster{cdb[]}[], "output cluster"=→"output cluster 2":T5)  [unwired: 5 in]
          }
          event "save(Logistic)": Value Change {
            n127 = event-data() -> ()  [unwired: 1 in, 6 out]
            n128 = local read "path (for logistic)"() -> (w517:path)
            n129 = local read "fitting (y&T)"() -> (w518:dbl[][])
            n130 = local read "Paramter guess"() -> (w520:dbl[])
            n131 = call "logistic save.vi"("file path (dialog if empty)"=w517, "format (%.3f)"="%.7e", "Paramter guess"=w520, "2D data"=w518) -> ()  [unwired: 10 in, 2 out]
          }
          event "x+": Value Change {
            w530 = u16 1 items=["Move X"=1, "Move Y"=2, "Single shot"=3, "single shot *15"=4, "energy adjustment"=5, "knife edge method"=6, "Auto mode"=7] ("Ring")
            n132 = event-data() -> ()  [unwired: 1 in, 6 out]
            n133 = local read "um(x)"() -> (w528:string)
            n134 = call "0814 labviewToEsp32.vi"("direction"="0", "um"=w528, "Ring"=w530) -> ("output"=w527:string)  [unwired: 8 in]
            n135 = VISA Write(VISA resource name=w526, write buffer=w527, error in (no error)=w525) -> (VISA resource name out=w524:refnum<visa-resource-name>, error out=w523:errorcluster)  [unwired: 1 out]
          }
          event "x-": Value Change {
            w540 = u16 1 items=["Move X"=1, "Move Y"=2, "Single shot"=3, "single shot *15"=4, "energy adjustment"=5, "knife edge method"=6, "Auto mode"=7] ("Ring")
            n136 = event-data() -> ()  [unwired: 1 in, 6 out]
            n137 = local read "um(x)"() -> (w538:string)
            n138 = call "0814 labviewToEsp32.vi"("direction"="1", "um"=w538, "Ring"=w540) -> ("output"=w537:string)  [unwired: 8 in]
            n139 = VISA Write(VISA resource name=w536, write buffer=w537, error in (no error)=w535) -> (VISA resource name out=w534:refnum<visa-resource-name>, error out=w533:errorcluster)  [unwired: 1 out]
          }
          event "y+": Value Change {
            w550 = u16 2 items=["Move X"=1, "Move Y"=2, "Single shot"=3, "single shot *15"=4, "energy adjustment"=5, "knife edge method"=6, "Auto mode"=7] ("Ring")
            n140 = event-data() -> ()  [unwired: 1 in, 6 out]
            n141 = local read "um(y)"() -> (w547:string)
            n142 = call "0814 labviewToEsp32.vi"("direction"="0", "um"=w547, "Ring"=w550) -> ("output"=w548:string)  [unwired: 8 in]
            n143 = VISA Write(VISA resource name=w546, write buffer=w548, error in (no error)=w545) -> (VISA resource name out=w544:refnum<visa-resource-name>, error out=w543:errorcluster)  [unwired: 1 out]
          }
          event "y-": Value Change {
            w560 = u16 2 items=["Move X"=1, "Move Y"=2, "Single shot"=3, "single shot *15"=4, "energy adjustment"=5, "knife edge method"=6, "Auto mode"=7] ("Ring")
            n144 = event-data() -> ()  [unwired: 1 in, 6 out]
            n145 = local read "um(y)"() -> (w551:string)
            n146 = call "0814 labviewToEsp32.vi"("direction"="1", "um"=w551, "Ring"=w560) -> ("output"=w558:string)  [unwired: 8 in]
            n147 = VISA Write(VISA resource name=w557, write buffer=w558, error in (no error)=w556) -> (VISA resource name out=w555:refnum<visa-resource-name>, error out=w554:errorcluster)  [unwired: 1 out]
          }
          event "knife edge method": Value Change {
            w570 = u16 6 items=["Move X"=1, "Move Y"=2, "Single shot"=3, "single shot *15"=4, "energy adjustment"=5, "knife edge method"=6, "Auto mode"=7] ("Ring")
            n148 = event-data() -> ()  [unwired: 1 in, 6 out]
            n149 = local read "um(x) 2"() -> (w566:string)
            n150 = local read "um/s"() -> (w565:string)
            n151 = call "0814 labviewToEsp32.vi"("scanspeed (um/s)"=w565, "um"=w566, "Ring"=w570) -> ("output"=w569:string)  [unwired: 8 in]
            n152 = VISA Write(VISA resource name=w568, write buffer=w569, error in (no error)=w567) -> (VISA resource name out=w562:refnum<visa-resource-name>, error out=w561:errorcluster)  [unwired: 1 out]
          }
          event "knife edge method(stop)": Value Change {
            w578 = u16 0 items=["Move X"=1, "Move Y"=2, "Single shot"=3, "single shot *15"=4, "energy adjustment"=5, "knife edge method"=6, "Auto mode"=7, "multiple shot"=8, "stop"=0] ("Ring")
            n153 = event-data() -> ()  [unwired: 1 in, 6 out]
            n154 = call "0814 labviewToEsp32.vi"("Ring"=w578) -> ("output"=w577:string)  [unwired: 10 in]
            n155 = VISA Write(VISA resource name=w576, write buffer=w577, error in (no error)=w575) -> (VISA resource name out=w572:refnum<visa-resource-name>, error out=w571:errorcluster)  [unwired: 1 out]
          }
        }
      }
      n156 = call "rsscope Initialize.vi"("VISA resource name"="VISA resource name", "ID Query (T: Check)"=TRUE, "Reset (T: Reset)"=FALSE) -> ("VISA resource name out"=w57:refnum<visa-resource-name>, "error out"=w58:errorcluster)  [unwired: 11 in]
      n157 = call "Get Channel Count"("instrument handle"=w57, "error in (no error)"=w58) -> ("instrument handle out"=w56:refnum<visa-resource-name>, "error out"=w51:errorcluster)  [unwired: 11 in, 1 out]
      n158 = property on="Tout" class="DigNum (strict)"("Value"=0 ("Tout")) -> (error out=w61:errorcluster)  [unwired: 2 in, 1 out]
      n159 = call "rsscope Configure Display Update.vi"("error in (no error)"=w51, "Display In Remote (Off)"=w55, "VISA resource name"=w56) -> ("error out"=w54:errorcluster, "VISA resource name out"=w53:refnum<visa-resource-name>)  [unwired: 7 in]
      n160 = while {
        tunnel: w61 -> [_]
        tunnel: [w100] -> _
        tunnel: w54 -> [w103]
        tunnel: w53 -> [w102]
        tunnel: [w101] -> w52
        stop <- w107 stop-if-true
        w104 = u8 0 ("Disabled")
        n161 = property on="Single" class="Bool"("Disabled"=w104) -> ()  [unwired: 2 in, 2 out]
        n162 = property on="Start" class="Bool"("Disabled"=w104) -> ()  [unwired: 2 in, 2 out]
        n163 = property on="timeout" class="DigNum (strict)"("Disabled"=w104) -> ()  [unwired: 2 in, 2 out]
        n164 = event shown="[0] \"Start\", \"Single\": Value Change" {
          selector: _ -> [_ _ _]
          dyn-events: _ -> [_ _ _]
          timeout: "Tout" -> [_ _ _]
          tunnel: [w117 _ w189] -> w101
          tunnel: w103 -> [w111 w181 w190]
          tunnel: [w116 w183 w190] -> w100
          tunnel: w102 -> [w112 w180 w189]
          tunnel: [_ _ "Exit"] -> w98
          event "Start", "Single": Value Change {
            w113 = u8 2 ("Disabled")
            n165 = event-data() -> ()  [unwired: 1 in, 1 out]
            n166 = property on="Stop" class="Bool"("Disabled"=u8 0) -> ()  [unwired: 2 in, 2 out]
            n167 = property on="Single" class="Bool"("Disabled"=w113) -> ()  [unwired: 2 in, 2 out]
            n168 = property on="timeout" class="DigNum (strict)"("Disabled"=w113) -> ()  [unwired: 2 in, 2 out]
            n169 = property on="Start" class="Bool"("Disabled"=w113) -> ()  [unwired: 2 in, 2 out]
            n170 = while {
              tunnel: "timeout" -> [w136]
              tunnel: [w134] -> w116
              tunnel: [w135] -> w117
              tunnel: w112 -> [w128]
              tunnel: w111 -> [w127]
              tunnel: "Single" -> [w126]
              shift-right: [w119] -> w109
              shift-left: dbl[] [] -> [w118]
              i -> [w132]
              stop <- w129 stop-if-true
              w124 = i32[] [1, 4] ("ActiveChannels")
              n171 = local read "Y(all)"() -> (w121:dbl[])
              n172 = Array Max & Min(array=w121) -> (max value=w120:dbl)  [unwired: 3 out]
              n173 = Build Array (concatenate)(w118, w120) -> (w119:dbl[])
              n174 = for {
                N: "channel on" -> [_]
                tunnel: w136 -> [w146]
                tunnel: [w145] -> w135
                tunnel: i8[] [1, 1] ("waveform") -> [w144] mode=indexing
                tunnel: w124 -> [w142] mode=indexing
                tunnel: [w141] -> w133 mode=indexing
                shift-right: [w143] -> w134
                shift-left: w127 -> [w147]
                tunnel: w128 -> [w138]
                tunnel: [w137] -> w125 mode=indexing
                i -> [w140]
                n175 = Equal To 0?(x=w140) -> (x = 0?=w139:bool)
                n176 = case shown="True" w139 {
                  tunnel: w147 -> [w167 w178]
                  tunnel: w146 -> [w166 _]
                  tunnel: [w165 w177] -> w145
                  tunnel: w144 -> [w164 w174]
                  tunnel: [w163 w173] -> w143
                  tunnel: w142 -> [w161 w172]
                  tunnel: [w162 w171] -> w141
                  tunnel: [w160 w168] -> w137
                  tunnel: w138 -> [w159 w170]
                  frame True {
                    n177 = call "rsscope Read Waveform.vi"("VISA resource name"=w159, "Waveform (1)"=w164, "Channel (1)"=w161, "Maximum Time (5000)"=w166, "error in (no error)"=w167) -> ("VISA resource name out"=w165:refnum<visa-resource-name>, "Waveform Array"=w155:dbl[], "Initial X"=w153:dbl, "X Increment"=w154:dbl, "error out"=w163:errorcluster)  [unwired: 6 in]
                    "Y(all)" <- w155
                    "X Increment" <- w154
                    "Initial X" <- w153
                    n178 = local read "X Increment"() -> (w149:dbl)
                    n179 = local read "Initial X"() -> (w148:dbl)
                    n180 = local read "T(all)"() -> (w152:dbl[])
                    n181 = local read "Y(all)"() -> (w151:dbl[])
                    n182 = Bundle("T(all)"=w152, "Y(all)"=w151, "X Increment"=w149, "Initial X"=w148) -> (→"output cluster":T6)  [unwired: 1 in]
                    n183 = call "data handle.vi"("unit"="unit", "Y"=w155, "X Increment (input)"=w154, "InitialX (input)"=w153) -> ("T"=w156:dbl[])  [unwired: 3 in, 3 out]
                    "T(all)" <- w156
                    n184 = Array Size(array=w155) -> (size(s)=w160:i32)
                    n185 = Bundle("Initial X"=w153, "X Increment"=w154, "Waveform Array"=w155) -> (w162:T18)  [unwired: 1 in]
                    n186 = Bundle("T"=w156, "Waveform Array"=w155) -> (→"waveform 1":cluster{"T":dbl[], "Waveform Array":dbl[]})  [unwired: 1 in]
                  }
                  frame False {
                    n187 = call "rsscope Fetch Waveform.vi"("Waveform (1)"=w174, "error in (no error)"=w178, "Channel (1)"=w172, "VISA resource name"=w170) -> ("error out"=w173:errorcluster, "Waveform Array"=w169:dbl[], "VISA resource name out"=w177:refnum<visa-resource-name>, "Initial X"=w175:dbl, "X Increment"=w176:dbl)  [unwired: 3 in]
                    n188 = Bundle("Initial X"=w175, "X Increment"=w176, "Waveform Array"=w169) -> (w171:T18)  [unwired: 1 in]
                    n189 = Array Size(array=w169) -> (size(s)=w168:i32)
                  }
                }
              }
              "Waveform" <- w133
              "Samples count" <- w125
              n190 = Unbundle By Name(w134) -> ("status"=w131:bool)
              n191 = Compound Arithmetic op=OR(w126, w131, "Stop") -> (w129:bool)
              "Acquisitions" <- w132
              "ActiveChannels" <- w124
            }
            "appended array" <- w109
          }
          event Timeout {
            n192 = event-data() -> ()  [unwired: 1 in, 2 out]
            n193 = local write "Tout"(-1 ("Tout")) -> ()
            n194 = for {
              N: 1 -> [_]
              tunnel: w180 -> [w188]
              shift-right: [w187] -> w183
              shift-left: w181 -> [w187]
              tunnel: [w186] -> _
              i -> [w184]
              n195 = call "Set Channel Enabled (CH1)"("instrument handle"=w188, "RepCap 'Channel' (CH1)"=w184, "Channel Enabled (OFF)"=TRUE) -> ("instrument handle out"=w186:refnum<visa-resource-name>)  [unwired: 11 in, 1 out]
            }
          }
          event "Exit": Value Change {
            n196 = event-data() -> ()  [unwired: 1 in, 1 out]
          }
        }
        n197 = property on="Stop" class="Bool"("Disabled"=u8 2) -> ()  [unwired: 2 in, 2 out]
        n198 = Unbundle By Name(w100) -> ("status"=w106:bool)
        n199 = Or(x=w106, y=w98) -> (x .or. y?=w107:bool)
      }
      n200 = while {
        tunnel: w90 -> [w245]
        tunnel: w89 -> [w244]
        tunnel: w84 -> [w243]
        shift-right: [w241] -> _
        shift-left: FALSE -> [w242]
        tunnel: [w240] -> w86
        tunnel: [w239] -> w85
        stop <- w247 stop-if-true
        n201 = property on="stop 2" class="Bool (strict)"() -> ("Value"=w238:bool)  [unwired: 2 in, 2 out]
        n202 = Dequeue Element(queue=w243, timeout in ms (-1)=50) -> (element=w249:T15, timed out?=w248:bool, error out=w252:errorcluster)  [unwired: 1 in, 1 out]
        n203 = Unbundle By Name(w252) -> ("status"=w251:bool)
        n204 = Or(x=w251, y=w238) -> (x .or. y?=w247:bool)
        n205 = case shown="False" w247 {
          tunnel: w244 -> [w259 w285]
          tunnel: w245 -> [w261 w286]
          tunnel: w249 -> [w255 _]
          tunnel: [w260 w286] -> w239
          tunnel: [w258 w285] -> w240
          tunnel: w248 -> [w257 _]
          tunnel: "Delay (ms)" -> [w256 _]
          tunnel: w242 -> [w254 w284]
          tunnel: [w253 w284] -> w241
          frame False {
            n206 = case shown="False" w257 {
              tunnel: w261 -> [w275 w283]
              tunnel: [w273 w283] -> w260
              tunnel: w259 -> [w274 w282]
              tunnel: [w272 w282] -> w258
              tunnel: w256 -> [w271 _]
              tunnel: w255 -> [w264 _]
              tunnel: w254 -> [w265 w281]
              tunnel: [w266 w281] -> w253
              frame False {
                w268 = u16 3 items=["MOVE", "HOME", "STOP", "Set Speed", "Info", "Set Zero"] ("Task")
                n207 = Unbundle By Name(w264) -> ("Task"=w263:u16)
                n208 = Equal?(x=w263, y=w268) -> (x = y?=w266:bool)
                n209 = Not(x=w266) -> (.not. x?=w267:bool)
                n210 = And(x=w265, y=w267) -> (x .and. y?=w262:bool)
                n211 = call "RS232 S&R 3.vi"("ReSetSPD"=w262, "error in"=w274, "Delay (ms)"=w271, "Stage Control"=w264, "VISA resource in"=w275) -> ("error out"=w272:errorcluster, "read"=w269:bool, "Cluster"=w270:T10, "VISA resource name out"=w273:refnum<visa-resource-name>)
                n212 = case shown="True" w269 {
                  tunnel: w270 -> [_ w280]
                  frame False {
                  }
                  frame True {
                    n213 = Unbundle By Name(w280) -> ("Current coordinates 2"=w278:cluster{"X":dbl, "Y":dbl, "Z":dbl})
                    "?" <- w278
                    n214 = Unbundle By Name(w280) -> ("Moving Time (Sec)"=→"Moving Time (Sec)":dbl)
                    n215 = feedback-in #1(w278) -> ()
                    n216 = feedback #1() -> (w277:cluster{"X":dbl, "Y":dbl, "Z":dbl})  [unwired: 1 in]
                    n217 = Equal?(x=w278, y=w277) -> (x = y?=→"Static":bool)
                    "Position Info" <- w280
                  }
                }
              }
              frame True {
              }
            }
          }
          frame True {
          }
        }
      }
      n218 = while {
        shift-right: [w196] -> w67
        shift-left: w64 -> [w198]
        shift-right: [w195] -> w66
        shift-left: w65 -> [w197]
        tunnel: w63 -> [w194]
        stop <- w193 stop-if-true
        n219 = case shown="True" "?" {
          tunnel: w198 -> [w199 w205]
          tunnel: w197 -> [w200 w204]
          tunnel: [w199 w203] -> w196
          tunnel: [w200 w202] -> w195
          tunnel: w194 -> [_ w201]
          frame False {
          }
          frame True {
            n220 = call <vilib>:"IMAQdx Grab.vi"("error in"=w204, "Image In"=w201, "Session In"=w205) -> ("error out"=w202:errorcluster, "Image Out"=w206:T3, "Session Out"=w203:T9)  [unwired: 1 in, 5 out]
            "Grab Image" <- w206
            n221 = case shown="True" "Get Image" {
              tunnel: w206 -> [_ w208]
              frame False {
              }
              frame True {
                "Snap Image" <- w208
              }
            }
          }
        }
        n222 = property on="stop 2" class="Bool (strict)"() -> ("Value"=w193:bool)  [unwired: 2 in, 2 out]
      }
      n223 = while {
        tunnel: w84 -> [w212]
        shift-right: [w210] -> _
        shift-left: 0 -> [w211]
        stop <- w209 stop-if-true
        w215 = 1000.0 ("value")
        w227 = u16 4 items=["MOVE", "HOME", "ZERO", "Set speed", "Info"] ("Ring")
        n224 = property on="Position to go" class="Clust (strict)"() -> ("Value"=w226:T8)  [unwired: 2 in, 2 out]
        n225 = Bundle("Ring"=w227, "Value"=w226) -> (w228:T19)  [unwired: 1 in]
        n226 = Enqueue Element(queue=w212, element=w228) -> (error out=w230:errorcluster)  [unwired: 2 in, 2 out]
        n227 = Unbundle By Name(w230) -> ("status"=w229:bool)
        n228 = property on="stop 2" class="Bool (strict)"() -> ("Value"=w231:bool)  [unwired: 2 in, 2 out]
        n229 = Or(x=w229, y=w231) -> (x .or. y?=w209:bool)
        n230 = case shown="False" w209 {
          frame False {
            n231 = Wait (ms)(milliseconds to wait="update period (ms)") -> ()  [unwired: 1 out]
          }
          frame True {
          }
        }
        n232 = property on="Moving Time (Sec)" class="DigNum (strict)"() -> ("Value"=w222:dbl)  [unwired: 2 in, 2 out]
        n233 = Tick Count (ms)() -> (millisecond timer value=w225:u32)
        n234 = First Call?() -> (First Call?: T/F=w224:bool)
        n235 = case shown="False" w224 {
          tunnel: w211 -> [w234 w235]
          tunnel: w225 -> [w233 w236]
          tunnel: [w233 w236] -> w210
          tunnel: [w232 w235] -> w223
          frame False {
            n236 = Subtract(x=w233, y=w234) -> (x-y=w232:u32)
          }
          frame True {
          }
        }
        n237 = Compound Arithmetic op=MULTIPLY(w215, w222) -> (w218:dbl)
        n238 = Not Equal To 0?(x=w218) -> (x != 0?=w214:bool)
        n239 = Subtract(x=w218, y=w223) -> (x-y=w220:dbl)
        n240 = Greater Than 0?(x=w220) -> (x > 0?=w219:bool)
        n241 = And(x=w219, y=w214) -> (x .and. y?=w213:bool)
        n242 = Select(t=w220, s=w213, f=0.0) -> (s? t:f=w216:dbl)
        n243 = Divide(x=w216, y=w215) -> (x/y=w217:dbl)
        n244 = property on="Moving Time (Sec)" class="DigNum (strict)"("Value"=w217) -> ()  [unwired: 2 in, 2 out]
      }
      n245 = call "rsscope Close.vi"("VISA resource name"=w52) -> ("error out"=w62:errorcluster)  [unwired: 10 in]
      n246 = call <vilib>:"Simple Error Handler.vi"("error in (no error)"=w62) -> ()  [unwired: 4 in, 5 out]
      n247 = call <vilib>:"IMAQdx Close Camera.vi"("error in"=w66, "Session In"=w67) -> ("error out"=w68:errorcluster)  [unwired: 9 out]
      n248 = call <vilib>:"Simple Error Handler.vi"("error in (no error)"=w68) -> ()  [unwired: 1 in, 8 out]
      n249 = VISA Close(VISA resource name=w78, error in (no error)=w77) -> ()  [unwired: 1 out]
      n250 = Release Queue(queue=w92, error in (no error)=w91) -> ()  [unwired: 1 in, 3 out]
      n251 = call "RS232 close.vi"("error in"=w86, "VISA resource name in"=w85) -> ("error out"=→"RS232 error":errorcluster)
    }
    frame #2 {
      n252 = property on="stop 2" class="Bool (strict)"("Value"=FALSE) -> ()  [unwired: 2 in, 2 out]
    }
  }
  n253 = local read "waveform 1"() -> (→"waveform 1":cluster{"T":dbl[], "Waveform Array":dbl[]})
